vi "Disconnect.vi"(7 "error in (no error)":errorcluster, 10 "Gantry In":refnum<k24>) -> (0 "error out":errorcluster)   [LabVIEW 2019, in "A3200.lvclass"]
uses:
  A3200.lvclass
  C:/Program Files (x86)/Aerotech/A3200/LabVIEW/2010/Bin/Aerotech.A3200.dll
  Program Files (x86)/Aerotech/A3200/LabVIEW/2010/Bin/Aerotech.A3200.dll
  Drivers/Aerotech A3200/Aerotech VIs.lvlib
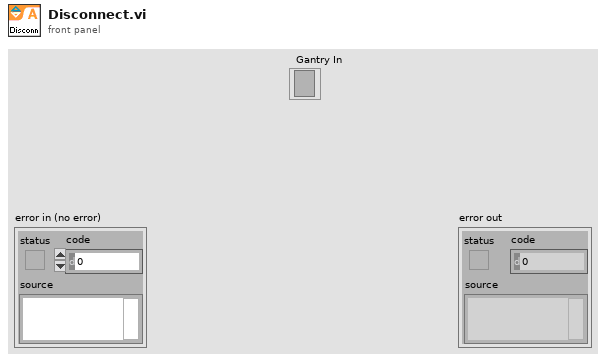
[diagram p1: front panel]
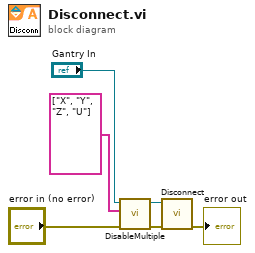
[diagram p0: block diagram]
diagram:
  n1 = call "DisableMultiple.vi"("error in (no error)"="error in (no error)", "axis names"=string[] ["X", "Y", "Z", "U"], "controller in"="Gantry In") -> ("error out"=w2:errorcluster, "controller out"=w5:refnum<k24>)  [unwired: 7 in]
  n2 = call "Disconnect.vi"("error in (no error)"=w2, "controller"=w5) -> ("error out"=→"error out":errorcluster)  [unwired: 9 in]
